vi "Untitled 2 (SubVI).vi"(11 "y":i32) -> (2 "Boolean":bool, 3 "Numeric":i32)   [LabVIEW 2015]
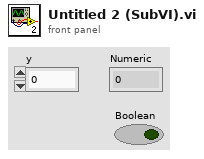
[diagram p1: front panel]
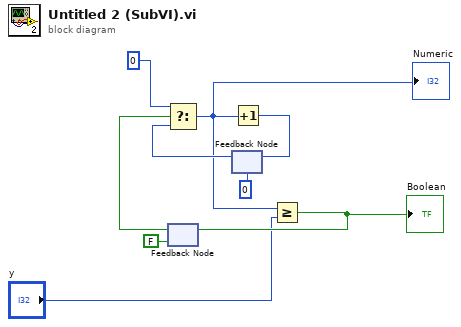
[diagram p0: block diagram]
diagram:
  n1 = feedback #1(FALSE) -> (w5:bool)
  n2 = feedback #2(0) -> (w9:i32)
  n3 = Select(t=0, s=w5, f=w9) -> (s? t:f=w1:i32)
  "Numeric" <- w1
  n4 = Increment(x=w1) -> (x+1=w7:i32)
  n5 = feedback-in #2(w7) -> ()
  n6 = Greater Or Equal?(x=w1, y="y") -> (x >= y?=w4:bool)
  "Boolean" <- w4
  n7 = feedback-in #1(w4) -> ()
